vi "Get Tab Test Result.vi"(8 "error in (no error)":errorcluster caption="entrée d'erreur (pas d'erreur)", 11 "Class Popup Result_Info (Virtual) en entrée":refnum<class "Class Popup Result_Info (Virtual).lvclass">) -> (0 "error out":errorcluster caption="sortie d'erreur", 2 "Tab Test Result":T3(array[cluster]), 3 "Class Popup Result_Info (Virtual) en sortie":refnum<class "Class Popup Result_Info (Virtual).lvclass">)   [LabVIEW 2020, in "Library Instrument & Equipement.lvlib" / "Library Popup.lvlib" / "Class Popup Result_Info (Virtual).lvclass"]
uses:
  Class Popup Result_Info (Virtual).lvclass
  Commun VI/TypeDef/Commande Test/Commande Value Type.ctl
  Commun VI/TypeDef/Commande Test/Commande Type Test.ctl
  Class Popup Result_Info (Virtual).lvclass/Class Popup Result_Info (Virtual).ctl
  Commun VI/Library Commun.lvlib
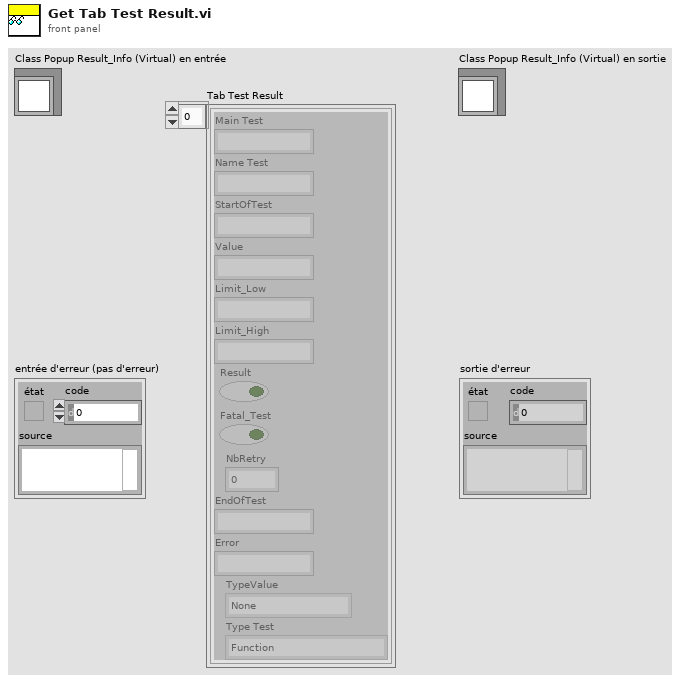
[diagram p1: front panel]
types:
  T1 = typedef "Library Commun.lvlib/Commande Value Type.ctl" = enum16{"None", "String", "Number", "Timestamp", "Boolean", "Array"}
  T2 = typedef "Library Commun.lvlib/Commande Type Test.ctl" = enum16{"Function", "Test", "Calculation"}
  T3 = cluster{"Main Test":string, "Name Test":string, "StartOfTest":string, "Value":string, "Limit_Low":string, "Limit_High":string, "Result":bool, "Fatal_Test":bool, "NbRetry":dbl, "EndOfTest":string, "Error":string, "TypeValue":T1, "Type Test":T2}[]
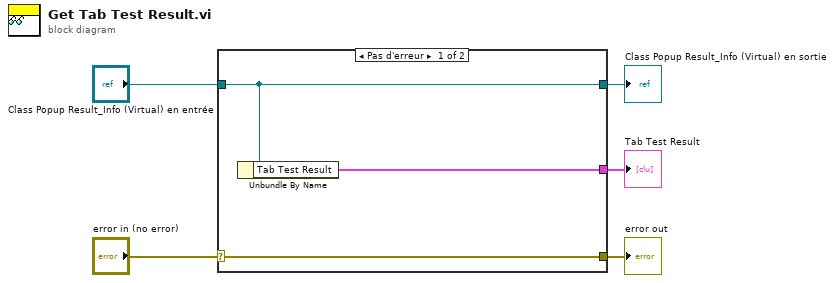
[diagram p0: block diagram]
diagram:
  n1 = case shown="Pas d'erreur" "error in (no error)" {
    selector: "error in (no error)" -> [w8 w9]
    tunnel: [w8 w9] -> w4
    tunnel: [w7 w10] -> w2
    tunnel: "Class Popup Result_Info (Virtual) en entrée" -> [w7 w10]
    tunnel: [w6 _] -> w1
    frame No Error {
      n2 = Unbundle By Name(w7) -> ("Tab Test Result"=w6:T3)
    }
    frame Error {
    }
  }
  "error out" <- w4
  "Class Popup Result_Info (Virtual) en sortie" <- w2
  "Tab Test Result" <- w1
